vi "OC2 Setup Alarm.vi"(3 "error in (no error)":errorcluster, 4 "alarm report in":T1 {"Temp limt Max" format="%.1f"; "Temp limt Min" format="%.1f"; "Temp ok max" format="%.2f"; "Temp ok min" format="%.2f"; "Alarm Max" format="%.2f"; "Alarm Min" format="%.2f"; "Alarms" items=["Off", "Min", "Max", "Both"]}, 5 "enable":bool, 6 "VISA resource name":refnum<visa-resource-name>) -> (0 "error out":errorcluster, 1 "alarm report out":T1 {"Temp limt Max" format="%.1f"; "Temp limt Min" format="%.1f"; "Temp ok max" format="%.2f"; "Temp ok min" format="%.2f"; "Alarm Max" format="%.2f"; "Alarm Min" format="%.2f"; "Alarms" items=["Off", "Min", "Max", "Both"]}, 2 "dup VISA resource name":refnum<visa-resource-name>)   [LabVIEW 2009]
doc: "TCM Setup Alarm.vi\n\nVI that sets the alarm information, accepts a cluster that contains the following variables:\nAlarms - of, min, max and both, reads which alarms are enabled\nAlarm min - minimum alarm temperature\nAlarm Max - maximum alarm value\nTemp ok min - \nTemp ok max - \nTemp limit min -\nTemp limit max -\n\nCOPYRIGHT ELECTRON DYNAMICS LTD"
panel:
  out "read data":string
  # "Set alarm variables"
  # "V1.02"
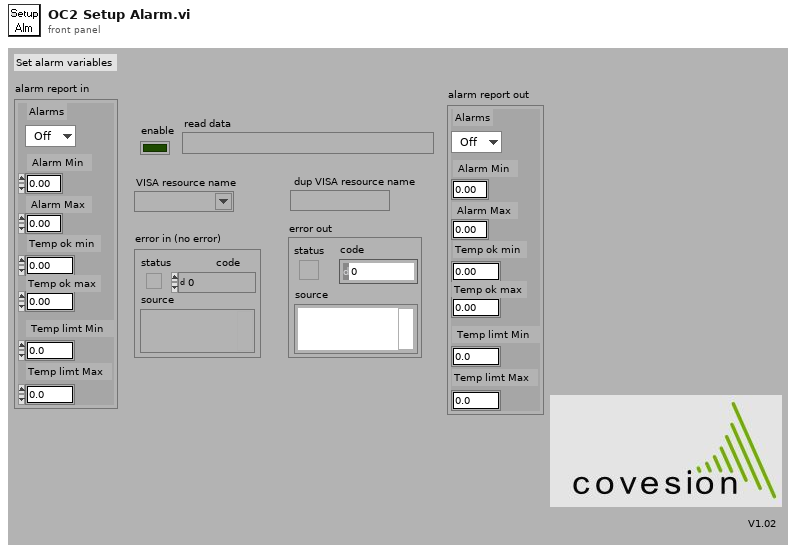
[diagram p1: front panel]
types:
  T1 = cluster{"Alarms":u16, " Alarm Min ":dbl, " Alarm Max ":dbl, "Temp ok min":dbl, "Temp ok max":dbl, " Temp limt Min ":dbl, "Temp limt Max ":dbl}
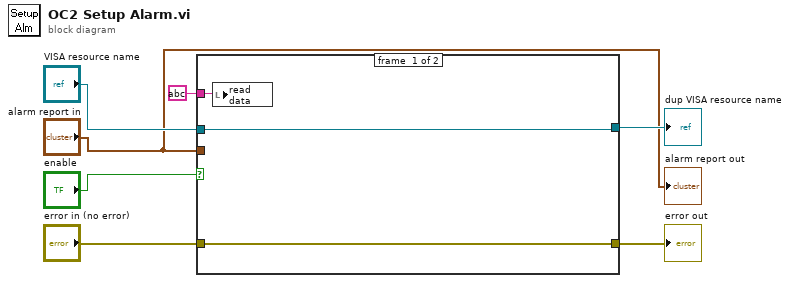
[diagram p0: block diagram]
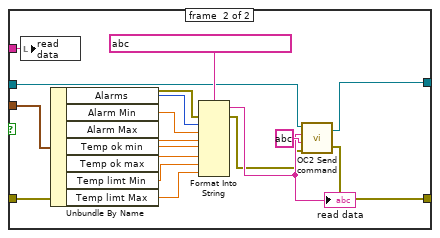
[diagram p2: hidden frame]
diagram:
  n1 = case shown="True" "enable" {
    tunnel: "alarm report in" -> [_ w24]
    tunnel: "VISA resource name" -> [w10 w14]
    tunnel: [w9 w13] -> w6
    tunnel: [w10 w12] -> w5
    tunnel: "error in (no error)" -> [w9 w16]
    tunnel: string ? -> [w8 w11]
    frame #0 {
      n2 = local write "read data"(w8) -> ()
    }
    frame #1 {
      n3 = local write "read data"(w11) -> ()
      n4 = Unbundle By Name(w24) -> ("Alarms"=w23:u16, "Alarm Min"=w22:dbl, "Alarm Max"=w21:dbl, "Temp ok min"=w20:dbl, "Temp ok max"=w19:dbl, "Temp limt Min"=w18:dbl, "Temp limt Max"=w17:dbl)
      n5 = Format Into String(format string=string ?, error in=w16, w23, w22, w21, w20, w19, w18, w17) -> (resulting string=w25:string, error out=w15:errorcluster)  [unwired: 1 in]
      "read data" <- w25
      n6 = call "OC2 Send command.vi"("VISA resource name"=w14, "Command data"=w25, "Command"=string ?, "error in (no error)"=w15) -> ("dup VISA resource name"=w12:refnum<visa-resource-name>, "error out"=w13:errorcluster)  [unwired: 1 in]
    }
  }
  "dup VISA resource name" <- w5
  "error out" <- w6
  "alarm report out" <- "alarm report in"
